vi "call header.vi"(8 "error in":errorcluster, 9 "Content String":string, 10 "Content-Length":i32, 11 "Host":string) -> (0 "error out":errorcluster, 3 "call string":string)   [LabVIEW 2009]
doc: "Prepends a Message Call Header to a message body"
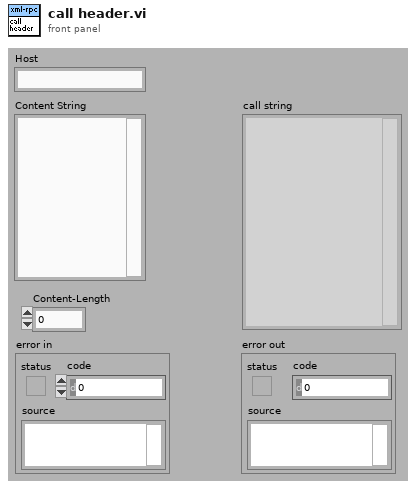
[diagram p1: front panel]
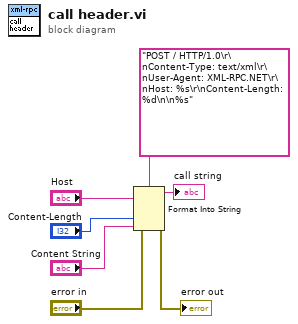
[diagram p0: block diagram]
diagram:
  n1 = Format Into String(format string="POST / HTTP/1.0\r\nContent-Type: text/xml\r\nUser-Agent: XML-RPC.NET\r\nHost: %s\r\nContent-Length: %d\n\n%s", error in="error in", "Host", "Content-Length", "Content String") -> (resulting string=→"call string":string, error out=→"error out":errorcluster)  [unwired: 1 in]
